vi "Sans titre 3.vi"(0 "Enable":bool=TRUE caption="Activer", 5 "error in (no error)":errorcluster caption="entrée d'erreur (pas d'erreur)") -> (15 "Adresse IP 3":string)   [LabVIEW 2019]
doc: "Affiche une boîte de dialogue standard qui invite l'utilisateur à entrer des informations, telles qu'un nom d'utilisateur et un mot de passe.\n--------------------\n\nCe VI Express est configuré comme suit :\n\nMessage à afficher à l'utilisateur :Adresse IP\nLes entrées sont : \nBoîte d'entrée de texte : Adresse IP"
panel:
  in  "Adresse IP":string
  out "error out":errorcluster caption="sortie d'erreur"
  out "String":string="Adresse IP" caption="Chaîne"
  in  "Cancel":bool caption="Annuler"
  in  "OK2":bool
  out "OK":bool
  in  "OK1":bool
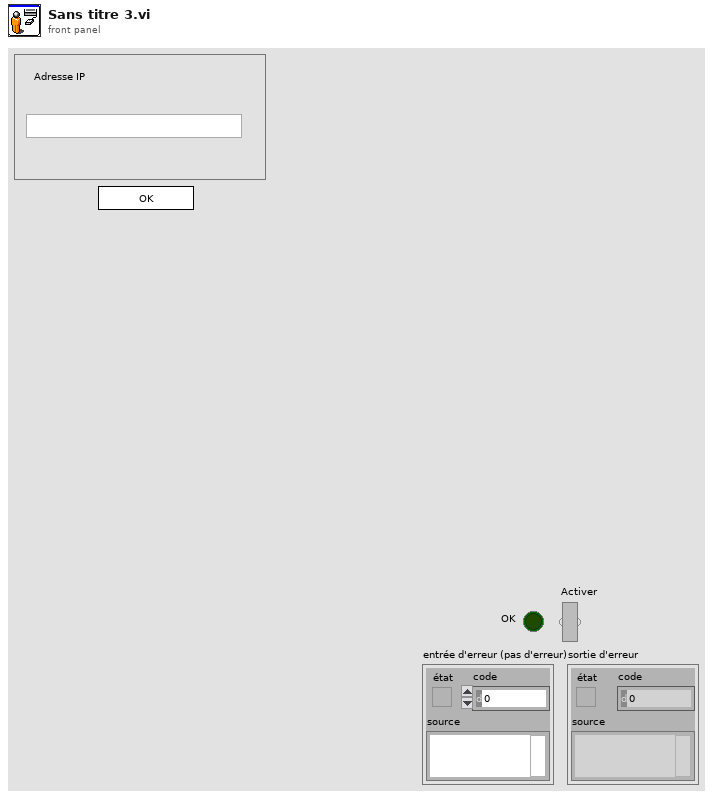
[diagram p1: front panel]
types:
  T1 = cluster{"Input Name":string, "Input Data Type":i32}[]
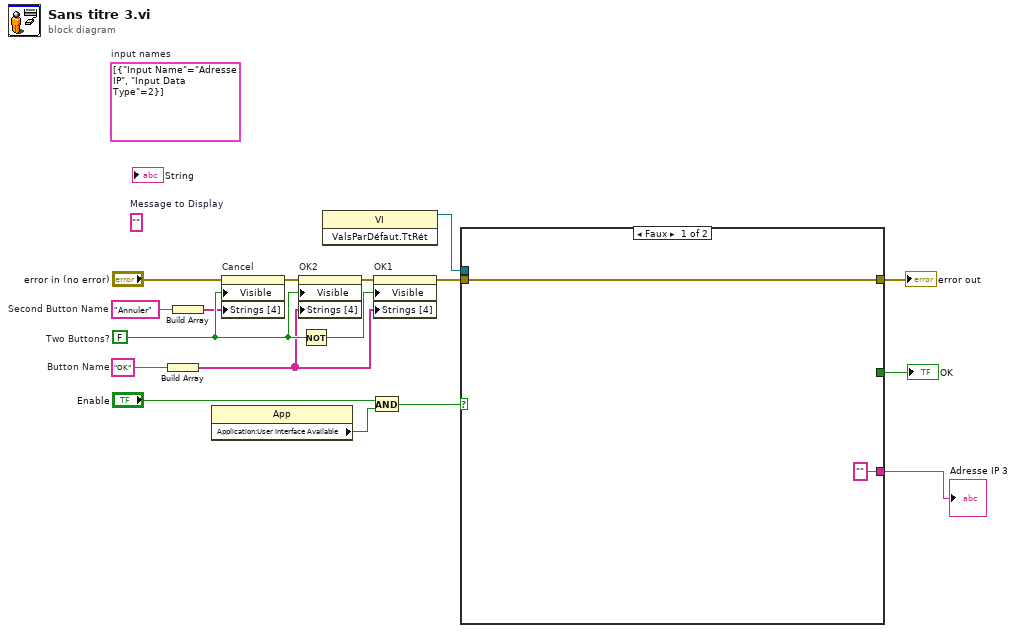
[diagram p0: block diagram]
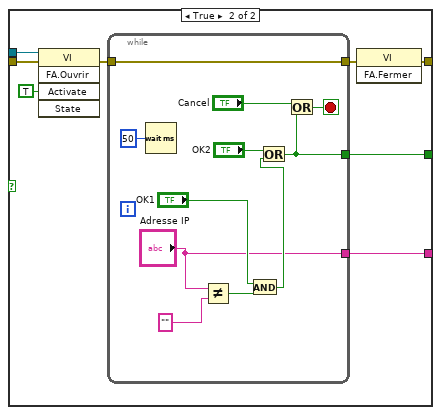
[diagram p2: hidden frame]
diagram:
  (unwired) T1 [{"Input Name"="Adresse IP", "Input Data Type"=2}]  # input names
  w11 = "Annuler"  # Second Button Name
  w9 = "OK"  # Button Name
  (unwired) ""  # Message to Display
  w17 = FALSE  # Two Buttons?
  n1 = Build Array(w9) -> (w10:string[])
  n2 = Build Array(w11) -> (w12:string[])
  n3 = property class="App"() -> ("Application:User Interface Available"=w4:bool)  [unwired: 2 in, 2 out]
  n4 = property on="Cancel" class="Bool"(error in="error in (no error)", "Visible"=w17, "Strings [4]"=w12) -> (error out=w14:errorcluster)  [unwired: 1 in, 1 out]
  n5 = property on="OK2" class="Bool"(error in=w14, "Visible"=w17, "Strings [4]"=w10) -> (error out=w13:errorcluster)  [unwired: 1 in, 1 out]
  n6 = Not(x=w17) -> (.not. x?=w15:bool)
  n7 = invoke class="VI" method="ValsParDéfaut.TtRét"() -> (reference out=w3:refnum<vi>)  [unwired: 3 in, 2 out]
  n8 = And(x="Enable", y=w4) -> (x .and. y?=w2:bool)
  n9 = property on="OK1" class="Bool"(error in=w13, "Visible"=w15, "Strings [4]"=w10) -> (error out=w8:errorcluster)  [unwired: 1 in, 1 out]
  n10 = case shown="Faux" w2 {
    tunnel: [_ w27] -> w16
    tunnel: w8 -> [w19 w26]
    tunnel: [w19 w25] -> w6
    tunnel: w3 -> [_ w24]
    tunnel: ["" ("Adresse IP") w20] -> w1
    frame False {
    }
    frame True {
      n11 = invoke class="VI" method="FA.Ouvrir"(reference=w24, error in=w26, "Activate"=TRUE ("Activate?")) -> (error out=w22:errorcluster)  [unwired: 2 in, 4 out]
      n12 = while "Main While Loop" {
        tunnel: [w35] -> w27
        tunnel: w22 -> [w33]
        tunnel: [w33] -> w21
        tunnel: ["Adresse IP"] -> w20
        stop <- w34 stop-if-true
        n13 = Wait (ms)(milliseconds to wait=u32 50 ("millisecond multiple")) -> ()  [unwired: 1 out]
        n14 = Not Equal?(x="Adresse IP", y="" ("Adresse IP")) -> (x != y?=w31:bool)
        n15 = And(x="OK1", y=w31) -> (x .and. y?=w29:bool)
        n16 = Or(x="OK2", y=w29) -> (x .or. y?=w35:bool)
        n17 = Or(x="Cancel", y=w35) -> (x .or. y?=w34:bool)
      }
      n18 = invoke class="VI" method="FA.Fermer"(error in=w21) -> (error out=w25:errorcluster)  [unwired: 2 in, 2 out]
    }
  }
  "OK" <- w16
  "error out" <- w6
  "Adresse IP 3" <- w1
